vi "Origin_Export_2014 05 02_JWa.vi"(6 "Input Conditions":T1, 7 "Analysis Array":string[][](array[string]), 8 "error in (no error)":errorcluster, 9 "Parameter Worksheet Name":string, 10 "Parameter Folder Script":string, 11 "Origin.IOApplication":refnum<k7>) -> (0 "error out":errorcluster, 2 "Origin.Worksheet":refnum<k7>, 3 "reference out":refnum<k7>)   [LabVIEW 2012]
panel:
  out "Dep Active Window":string
  out "Indep Unit":string
  out "Dep Unit":string
  out "Dep Used":string
  out "Indep Used":string
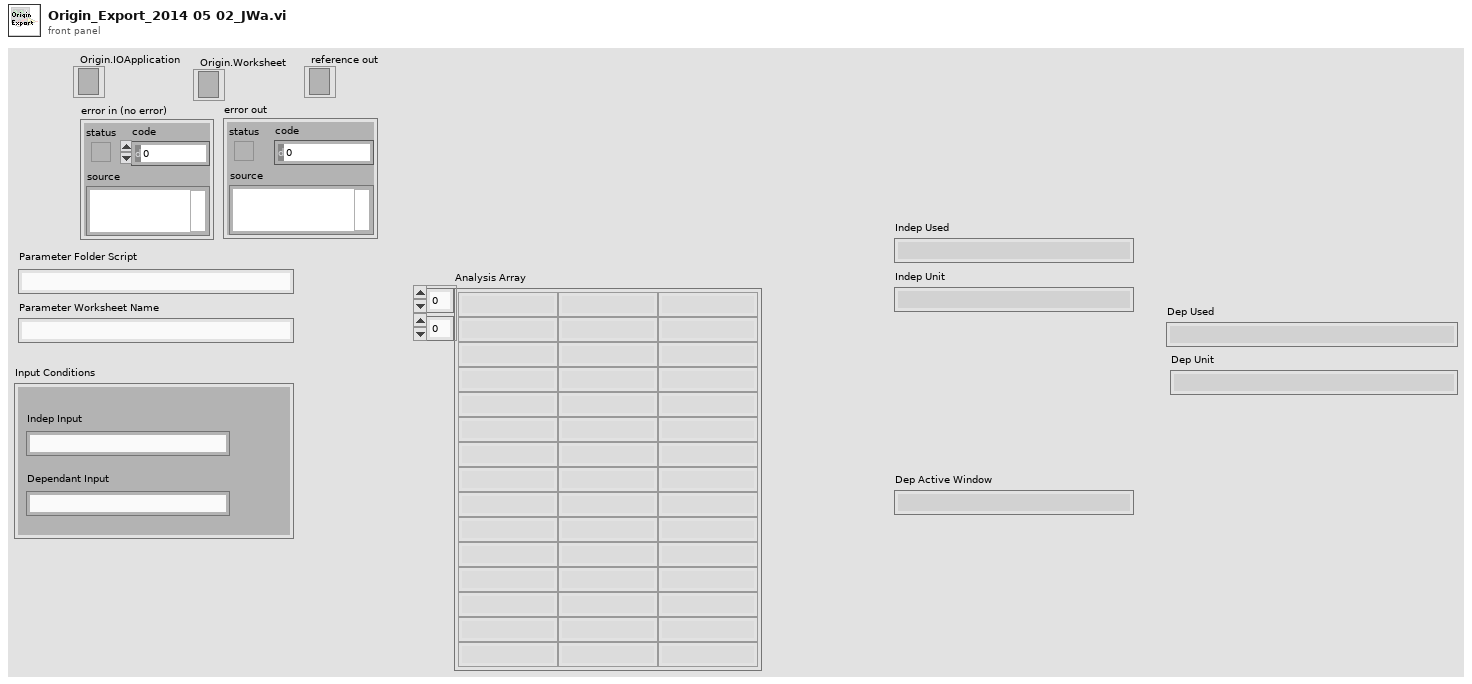
[diagram p1: front panel]
types:
  T1 = cluster{"Indep Input":string, "Dependant Input":string}
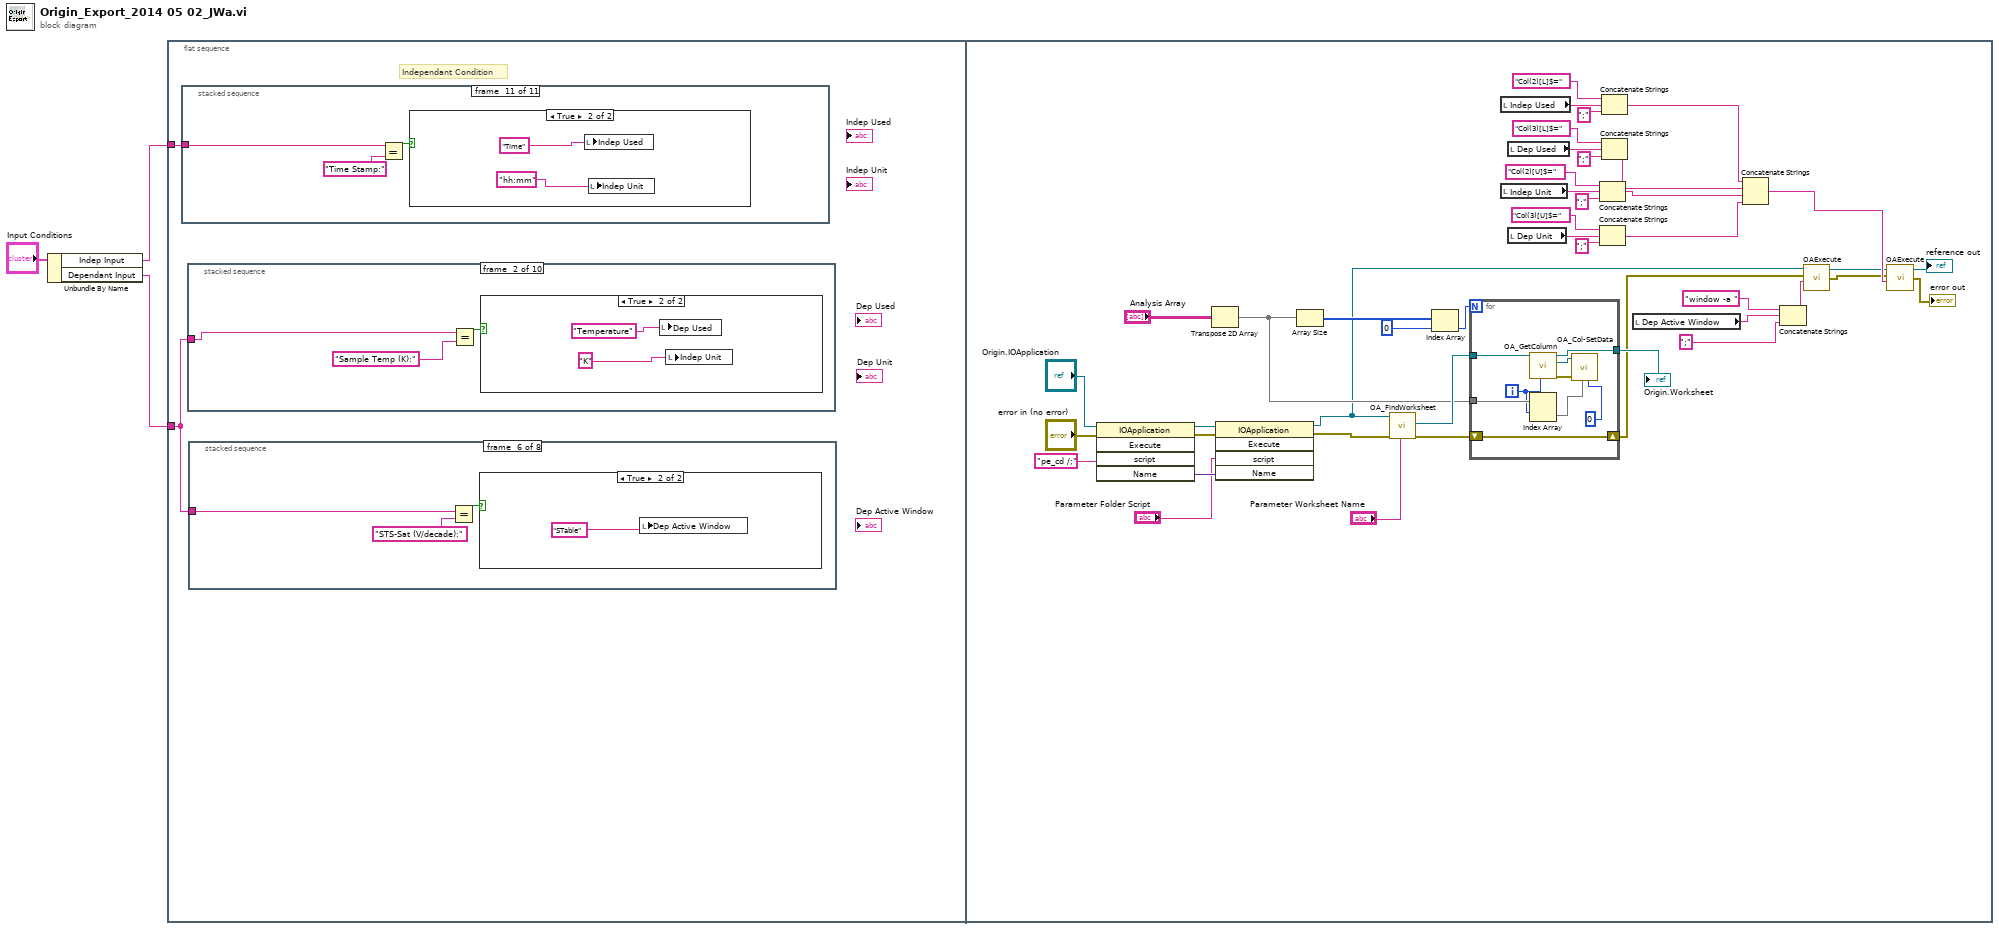
[diagram p0: block diagram]
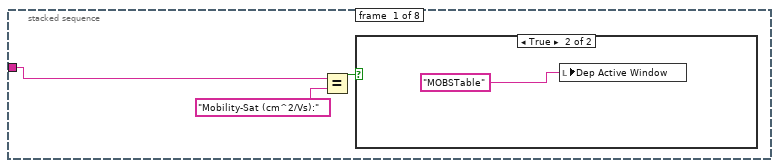
[diagram p2: hidden frame]
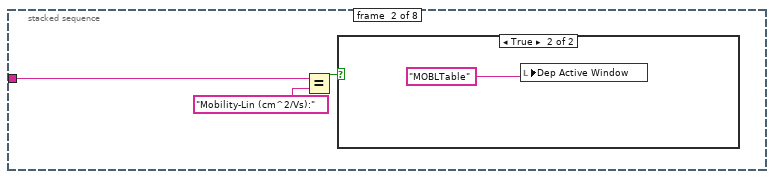
[diagram p4: hidden frame]
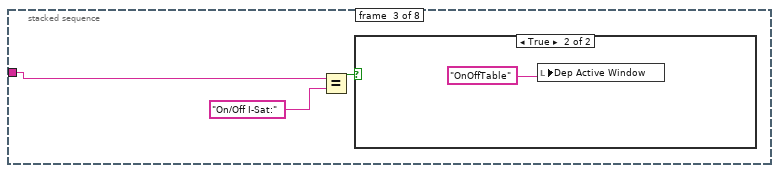
[diagram p6: hidden frame]
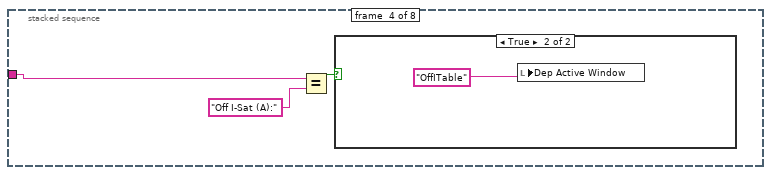
[diagram p8: hidden frame]
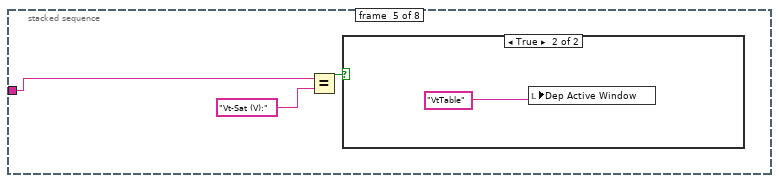
[diagram p10: hidden frame]
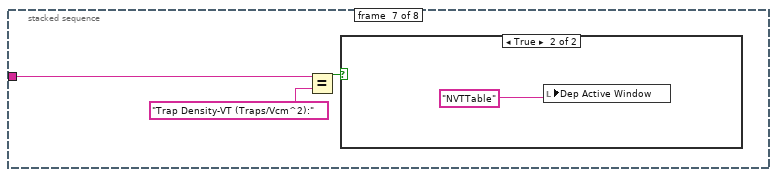
[diagram p13: hidden frame]
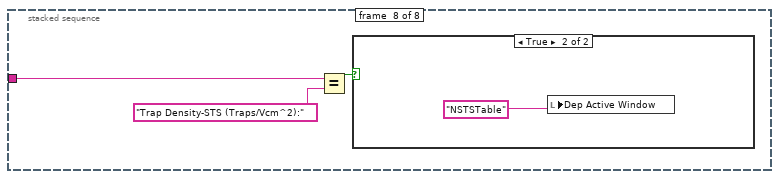
[diagram p15: hidden frame]
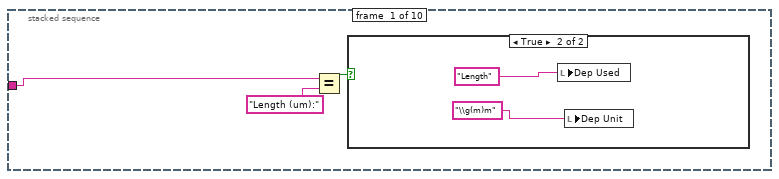
[diagram p17: hidden frame]
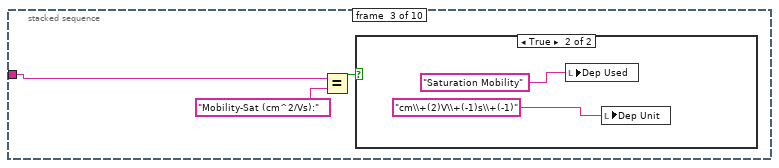
[diagram p20: hidden frame]
diagram:
  n1 = Unbundle By Name("Input Conditions") -> ("Indep Input"=w2:string, "Dependant Input"=w1:string)
  n2 = flat-sequence {
    tunnel: w2 -> [w5]
    tunnel: w1 -> [w4]
    frame #0 {
      # "Independant Condition"
      n3 = stacked-sequence {
        tunnel: w5 -> [w88 w93 w98 w103 w108 w113 w118 w123 w128 w133 w138]
        frame #0 {
          n4 = Equal?(x=w88, y="Length (um):") -> (x = y?=w89:bool)
          n5 = case shown="True" w89 {
            frame False {
            }
            frame True {
              n6 = local write "Indep Used"("Length") -> ()
              n7 = local write "Indep Unit"("\\g(m)m") -> ()
            }
          }
        }
        frame #1 {
          n8 = Equal?(x=w93, y="Sample Temp (K):") -> (x = y?=w94:bool)
          n9 = case shown="True" w94 {
            frame False {
            }
            frame True {
              n10 = local write "Indep Used"("Temperature") -> ()
              n11 = local write "Indep Unit"("K") -> ()
            }
          }
        }
        frame #2 {
          n12 = Equal?(x=w98, y="Mobility-Sat (cm^2/Vs):") -> (x = y?=w99:bool)
          n13 = case shown="True" w99 {
            frame False {
            }
            frame True {
              n14 = local write "Indep Used"("Saturation Mobility") -> ()
              n15 = local write "Indep Unit"("cm\\+(2)V\\+(-1)s\\+(-1)") -> ()
            }
          }
        }
        frame #3 {
          n16 = Equal?(x=w103, y="Mobility-Lin (cm^2/Vs):") -> (x = y?=w104:bool)
          n17 = case shown="True" w104 {
            frame False {
            }
            frame True {
              n18 = local write "Indep Used"("Linear Mobility") -> ()
              n19 = local write "Indep Unit"("cm\\+(2)V\\+(-1)s\\+(-1)") -> ()
            }
          }
        }
        frame #4 {
          n20 = Equal?(x=w108, y="On/Off I-Sat:") -> (x = y?=w109:bool)
          n21 = case shown="True" w109 {
            frame False {
            }
            frame True {
              n22 = local write "Indep Used"("On/Off Current") -> ()
              n23 = local write "Indep Unit"("") -> ()
            }
          }
        }
        frame #5 {
          n24 = Equal?(x=w113, y="Off I-Sat (A):") -> (x = y?=w114:bool)
          n25 = case shown="True" w114 {
            frame False {
            }
            frame True {
              n26 = local write "Indep Used"("Off Current") -> ()
              n27 = local write "Indep Unit"("A") -> ()
            }
          }
        }
        frame #6 {
          n28 = Equal?(x=w118, y="Vt-Sat (V):") -> (x = y?=w119:bool)
          n29 = case shown="True" w119 {
            frame False {
            }
            frame True {
              n30 = local write "Indep Used"("Threshold Voltage") -> ()
              n31 = local write "Indep Unit"("V") -> ()
            }
          }
        }
        frame #7 {
          n32 = Equal?(x=w123, y="STS-Sat (V/decade):") -> (x = y?=w124:bool)
          n33 = case shown="True" w124 {
            frame False {
            }
            frame True {
              n34 = local write "Indep Used"("STS") -> ()
              n35 = local write "Indep Unit"("V dec\\+(-1)") -> ()
            }
          }
        }
        frame #8 {
          n36 = Equal?(x=w128, y="Trap Density-VT (Traps/Vcm^2):") -> (x = y?=w129:bool)
          n37 = case shown="True" w129 {
            frame False {
            }
            frame True {
              n38 = local write "Indep Used"("Trap Density-VT") -> ()
              n39 = local write "Indep Unit"("Traps V\\+(-1)cm\\+(-2)\\+()\\+()") -> ()
            }
          }
        }
        frame #9 {
          n40 = Equal?(x=w133, y="Trap Density-STS (Traps/Vcm^2):") -> (x = y?=w134:bool)
          n41 = case shown="True" w134 {
            frame False {
            }
            frame True {
              n42 = local write "Indep Used"("Trap Density-STS") -> ()
              n43 = local write "Indep Unit"("Traps V\\+(-1)cm\\+(-2)\\+()\\+()") -> ()
            }
          }
        }
        frame #10 {
          n44 = Equal?(x=w138, y="Time Stamp:") -> (x = y?=w139:bool)
          n45 = case shown="True" w139 {
            frame False {
            }
            frame True {
              n46 = local write "Indep Used"("Time") -> ()
              n47 = local write "Indep Unit"("hh:mm") -> ()
            }
          }
        }
      }
      n48 = stacked-sequence {
        tunnel: w4 -> [w38 w43 w48 w53 w58 w63 w68 w73 w78 w83]
        frame #0 {
          n49 = Equal?(x=w38, y="Length (um):") -> (x = y?=w39:bool)
          n50 = case shown="True" w39 {
            frame False {
            }
            frame True {
              n51 = local write "Dep Used"("Length") -> ()
              n52 = local write "Dep Unit"("\\g(m)m") -> ()
            }
          }
        }
        frame #1 {
          n53 = Equal?(x=w43, y="Sample Temp (K):") -> (x = y?=w44:bool)
          n54 = case shown="True" w44 {
            frame False {
            }
            frame True {
              n55 = local write "Dep Used"("Temperature") -> ()
              n56 = local write "Indep Unit"("K") -> ()
            }
          }
        }
        frame #2 {
          n57 = Equal?(x=w48, y="Mobility-Sat (cm^2/Vs):") -> (x = y?=w49:bool)
          n58 = case shown="True" w49 {
            frame False {
            }
            frame True {
              n59 = local write "Dep Used"("Saturation Mobility") -> ()
              n60 = local write "Dep Unit"("cm\\+(2)V\\+(-1)s\\+(-1)") -> ()
            }
          }
        }
        frame #3 {
          n61 = Equal?(x=w53, y="Mobility-Lin (cm^2/Vs):") -> (x = y?=w54:bool)
          n62 = case shown="True" w54 {
            frame False {
            }
            frame True {
              n63 = local write "Dep Used"("Linear Mobility") -> ()
              n64 = local write "Dep Unit"("cm\\+(2)V\\+(-1)s\\+(-1)") -> ()
            }
          }
        }
        frame #4 {
          n65 = Equal?(x=w58, y="On/Off I-Sat:") -> (x = y?=w59:bool)
          n66 = case shown="True" w59 {
            frame False {
            }
            frame True {
              n67 = local write "Dep Unit"("") -> ()
              n68 = local write "Dep Used"("On/Off Current") -> ()
            }
          }
        }
        frame #5 {
          n69 = Equal?(x=w63, y="Off I-Sat (A):") -> (x = y?=w64:bool)
          n70 = case shown="True" w64 {
            frame False {
            }
            frame True {
              n71 = local write "Dep Unit"("A") -> ()
              n72 = local write "Dep Used"("Off Current") -> ()
            }
          }
        }
        frame #6 {
          n73 = Equal?(x=w68, y="Vt-Sat (V):") -> (x = y?=w69:bool)
          n74 = case shown="True" w69 {
            frame False {
            }
            frame True {
              n75 = local write "Dep Used"("Threshold Voltage") -> ()
              n76 = local write "Dep Unit"("V") -> ()
            }
          }
        }
        frame #7 {
          n77 = Equal?(x=w73, y="STS-Sat (V/decade):") -> (x = y?=w74:bool)
          n78 = case shown="True" w74 {
            frame False {
            }
            frame True {
              n79 = local write "Dep Used"("STS") -> ()
              n80 = local write "Dep Unit"("V dec\\+(-1)") -> ()
            }
          }
        }
        frame #8 {
          n81 = Equal?(x=w78, y="Trap Density-VT (Traps/Vcm^2):") -> (x = y?=w79:bool)
          n82 = case shown="True" w79 {
            frame False {
            }
            frame True {
              n83 = local write "Dep Used"("Trap Density-VT") -> ()
              n84 = local write "Dep Unit"("Traps V\\+(-1)cm\\+(-2)\\+()\\+()") -> ()
            }
          }
        }
        frame #9 {
          n85 = Equal?(x=w83, y="Trap Density-STS (Traps/Vcm^2):") -> (x = y?=w84:bool)
          n86 = case shown="True" w84 {
            frame False {
            }
            frame True {
              n87 = local write "Dep Used"("Trap Density-STS") -> ()
              n88 = local write "Dep Unit"("Traps V\\+(-1)cm\\+(-2)\\+()\\+()") -> ()
            }
          }
        }
      }
      n89 = stacked-sequence {
        tunnel: w4 -> [w6 w10 w14 w18 w22 w26 w30 w34]
        frame #0 {
          n90 = Equal?(x=w6, y="Mobility-Sat (cm^2/Vs):") -> (x = y?=w7:bool)
          n91 = case shown="True" w7 {
            frame False {
            }
            frame True {
              n92 = local write "Dep Active Window"("MOBSTable") -> ()
            }
          }
        }
        frame #1 {
          n93 = Equal?(x=w10, y="Mobility-Lin (cm^2/Vs):") -> (x = y?=w11:bool)
          n94 = case shown="True" w11 {
            frame False {
            }
            frame True {
              n95 = local write "Dep Active Window"("MOBLTable") -> ()
            }
          }
        }
        frame #2 {
          n96 = Equal?(x=w14, y="On/Off I-Sat:") -> (x = y?=w15:bool)
          n97 = case shown="True" w15 {
            frame False {
            }
            frame True {
              n98 = local write "Dep Active Window"("OnOffTable") -> ()
            }
          }
        }
        frame #3 {
          n99 = Equal?(x=w18, y="Off I-Sat (A):") -> (x = y?=w19:bool)
          n100 = case shown="True" w19 {
            frame False {
            }
            frame True {
              n101 = local write "Dep Active Window"("OffITable") -> ()
            }
          }
        }
        frame #4 {
          n102 = Equal?(x=w22, y="Vt-Sat (V):") -> (x = y?=w23:bool)
          n103 = case shown="True" w23 {
            frame False {
            }
            frame True {
              n104 = local write "Dep Active Window"("VtTable") -> ()
            }
          }
        }
        frame #5 {
          n105 = Equal?(x=w26, y="STS-Sat (V/decade):") -> (x = y?=w27:bool)
          n106 = case shown="True" w27 {
            frame False {
            }
            frame True {
              n107 = local write "Dep Active Window"("STable") -> ()
            }
          }
        }
        frame #6 {
          n108 = Equal?(x=w30, y="Trap Density-VT (Traps/Vcm^2):") -> (x = y?=w31:bool)
          n109 = case shown="True" w31 {
            frame False {
            }
            frame True {
              n110 = local write "Dep Active Window"("NVTTable") -> ()
            }
          }
        }
        frame #7 {
          n111 = Equal?(x=w34, y="Trap Density-STS (Traps/Vcm^2):") -> (x = y?=w35:bool)
          n112 = case shown="True" w35 {
            frame False {
            }
            frame True {
              n113 = local write "Dep Active Window"("NSTSTable") -> ()
            }
          }
        }
      }
    }
    frame #1 {
      n114 = invoke class="IOApplication" method="Execute"(reference="Origin.IOApplication", error in="error in (no error)", "script"="pe_cd /;") -> (reference out=w185:refnum<k7>, error out=w184:errorcluster, "Name"=w183:variant)  [unwired: 2 in, 2 out]
      n115 = Transpose 2D Array(2D array="Analysis Array") -> (transposed array=w176:string[][])
      n116 = invoke class="IOApplication" method="Execute"(reference=w185, error in=w184, "script"="Parameter Folder Script", "Name"=w183) -> (reference out=w150:refnum<k7>, error out=w172:errorcluster)  [unwired: 1 in, 3 out]
      n117 = Array Size(array=w176) -> (size(s)=w180:i32[])
      n118 = call "OA_FindWorksheet.vi"("Name"="Parameter Worksheet Name", "error in (no error)"=w172, "Origin.IOApplication"=w150) -> ("error out"=w181:errorcluster, "Origin.Worksheet"=w182:refnum<k7>)  [unwired: 6 in, 1 out]
      n119 = Index Array(array=w180, index=0) -> (element=w179:i32)
      n120 = for {
        N: w179 -> [_]
        tunnel: w182 -> [w195]
        tunnel: w176 -> [w194]
        tunnel: [w193] -> w177
        shift-right: [w189] -> w152
        shift-left: w181 -> [w189]
        i -> [w188]
        n121 = call "OA_GetColumn.vi"("Column Name/Index"=w188, "Origin.Worksheet"=w195) -> ("error out"=w191:errorcluster, "Origin.Column"=w192:refnum<k7>, "Origin.Worksheet"=w193:refnum<k7>)  [unwired: 7 in]
        n122 = Index Array(array=w194, index (row)=w188) -> (element=w190:string[])  [unwired: 1 in]
        n123 = call "OA_Col-SetData.vi"("Origin.Column"=w192, "error in (no error)"=w191, "data"=w190, "nOffset"=0) -> ()  [unwired: 3 in, 3 out]
      }
      "Origin.Worksheet" <- w177
      n124 = local read "Indep Used"() -> (w156:string)
      n125 = local read "Indep Unit"() -> (w161:string)
      n126 = local read "Dep Used"() -> (w157:string)
      n127 = local read "Dep Unit"() -> (w162:string)
      n128 = Concatenate Strings("Col(2)[U]$=", w161, ";") -> (w159:string)
      n129 = Concatenate Strings("Col(3)[U]$=", w162, ";") -> (w158:string)
      n130 = Concatenate Strings("Col(2)[L]$=", w156, ";") -> (w153:string)
      n131 = Concatenate Strings("Col(3)[L]$=", w157, ";") -> (w155:string)
      n132 = local read "Dep Active Window"() -> (w147:string)
      n133 = Concatenate Strings(w153, w155, w159, w158) -> (w154:string)
      n134 = Concatenate Strings("window -a ", w147, ";") -> (w145:string)
      n135 = call "OAExecute.vi"("script"=w145, "Error IO"=w152, "Origin.IOApplication"=w150) -> ("Error IO Out"=w151:errorcluster, "Origin.IOApplication"=w149:refnum<k7>)  [unwired: 1 in, 1 out]
      n136 = call "OAExecute.vi"("script"=w154, "Error IO"=w151, "Origin.IOApplication"=w149) -> ("Error IO Out"=→"error out":errorcluster, "Origin.IOApplication"=→"reference out":refnum<k7>)  [unwired: 1 in, 1 out]
    }
  }
